vi "configure generador FULL_standalone.vi"(8 "error in":errorcluster, 9 "Amplitude (1.0 Vpp)":dbl=1.0, 10 "Config Pulse":T1={"Channel"=1, "Frequency"=1000000.001, "Width Time"=3.3e-09, "Amplitude"=0.3, "DC Offset"=0.0, "Load"=50.0, "Leading Edge Time"=1e-09, "Trailing Edge Time"=1e-09, "Delay"=0.0, "Out"=TRUE, "/Out"=TRUE, "Trigger Level Sync"=0, "Trigger Sync Out"=0, "Vasic Theorical"=50.0} {"Vasic Theorical" min=1.0 max=1000000.0 step=1.0 format="%#_6pV"; "Frequency" min=0.001 max=333000000.0 step=1000.0 format="%#_6pHz"; "Leading Edge Time" min=1e-09 max=1.0 step=1e-10 format="%#_6ps"; "Trailing Edge Time" min=1e-09 max=1.0 step=1e-10 format="%#_6ps"; "Delay" min=0.0 max=1.0 step=1e-12 format="%#_6ps"; "Trigger Level Sync" items=["ECL", "TTL"]; "Trigger Sync Out" items=["AB"=3, "B"=2, "A"=1, "None"=0]; "Load" min=1.0 max=1000000.0 step=1.0 format="%#_6p"; "DC Offset" min=-10.0 max=10.0 step=0.1 format="%#_6pV"; "Amplitude" min=0.05 max=5.0 step=0.001 format="%#_6pV"; "Width Time" min=1.5e-09 max=1.0 step=1e-10 format="%#_6ps"; "Channel" items=["Channel1"=1, "Channel2"=2]}, 11 "VISA Key 81160A":refnum<visa-resource-name>="USB0::0x0957::0x4108::MY51400682::INSTR") -> (0 "error out":errorcluster, 2 "Amplitude":dbl=0.3, 3 "VISA Key 81160A 2":refnum<visa-resource-name>="USB0::0x0957::0x4108::MY51400682::INSTR")   [LabVIEW 2019]
uses:
  GenPulse_configurar.ctl
  Viejos/Alfredo LABVIEW/Set-up verificador ASICs/Lib Agilent 81160A/Agilent 81150/Agilent 81150.lvlib
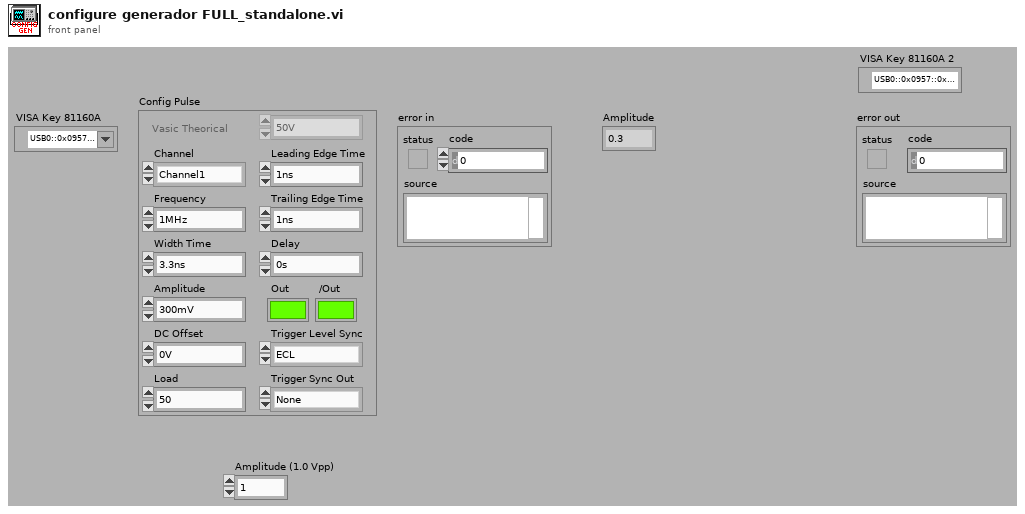
[diagram p1: front panel]
types:
  T1 = typedef "GenPulse_configurar.ctl" = cluster{"Channel":u16, "Frequency":dbl, "Width Time":dbl, "Amplitude":dbl, "DC Offset":dbl, "Load":dbl, "Leading Edge Time":dbl, "Trailing Edge Time":dbl, "Delay":dbl, "Out":bool, "/Out":bool, "Trigger Level Sync":u16, "Trigger Sync Out":u16, "Vasic Theorical":dbl}
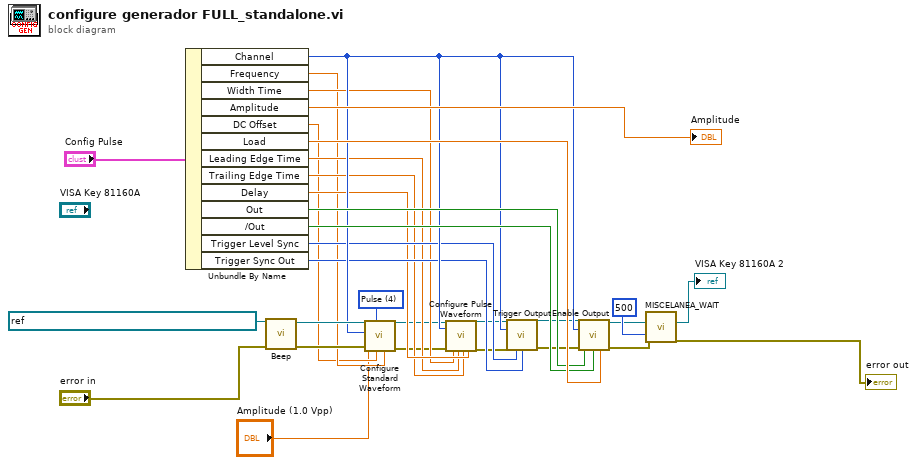
[diagram p0: block diagram]
diagram:
  w6 = u16 4 items=["Sine", "Square", "Ramp Up", "Ramp Down", "Pulse", "Noise", "DC"] ("Waveform (0: Sine)")
  n1 = Unbundle By Name("Config Pulse") -> ("Channel"=w21:u16, "Frequency"=w8:dbl, "Width Time"=w11:dbl, "Amplitude"=→"Amplitude":dbl, "DC Offset"=w7:dbl, "Load"=w24:dbl, "Leading Edge Time"=w12:dbl, "Trailing Edge Time"=w13:dbl, "Delay"=w14:dbl, "Out"=w22:bool, "/Out"=w23:bool, "Trigger Level Sync"=w17:u16, "Trigger Sync Out"=w18:u16)
  n2 = call "Beep.vi"("VISA resource name"=refnum<visa-resource-name> "USB0::0x0957::0x4108::MY51400682::INSTR", "error in (no error)"="error in") -> ("VISA resource name out"=w27:refnum<visa-resource-name>, "error out"=w26:errorcluster)  [unwired: 12 in]
  n3 = call "Configure Standard Waveform.vi"("Frequency (1000.0 Hz)"=w8, "DC Offset (0.0 Volts)"=w7, "Waveform (0: Sine)"=w6, "error in (no error)"=w26, "Amplitude (1.0 Vpp)"="Amplitude (1.0 Vpp)", "Channel (1: Channel1)"=w21, "VISA resource name"=w27) -> ("error out"=w10:errorcluster, "VISA resource name out"=w9:refnum<visa-resource-name>)  [unwired: 3 in]
  n4 = call "Configure Pulse Waveform.vi"("VISA resource name"=w9, "Channel (1: Channel1)"=w21, "error in (no error)"=w10, "Width (1.5E-9 Sec)"=w11, "Leading Edge Time\n(1.0E-9 Sec)"=w12, "Trailing Edge Time\n(1.0E-9 Sec)"=w13, "Delay\n(0.0 Seconds)"=w14) -> ("VISA resource name out"=w15:refnum<visa-resource-name>, "error out"=w16:errorcluster)  [unwired: 11 in]
  n5 = call "Trigger Output.vi"("VISA resource name"=w15, "Channel (1: Channel1)"=w21, "error in (no error)"=w16, "Trigger Sync Out (1: A)"=w17, "Trigger Level Sync (0: ECL)"=w18) -> ("VISA resource name out"=w19:refnum<visa-resource-name>, "error out"=w20:errorcluster)  [unwired: 9 in]
  n6 = call "Enable Output.vi"("VISA resource name"=w19, "Channel (1: Channel1)"=w21, "error in (no error)"=w20, "Enable Output (T: Enable)"=w22, "Enable Output Complement (T: Enable)"=w23, "Load (50 Ohm)"=w24) -> ("VISA resource name out"=→"VISA Key 81160A 2":refnum<visa-resource-name>, "error out"=w28:errorcluster)  [unwired: 8 in]
  n7 = call "MISCELANEA_WAIT.vi"("ms wait IN"=u32 500, "Error IN"=w28) -> ("Error OUT"=→"error out":errorcluster)  [unwired: 16 in, 1 out]
